vi "Oscilloscope_Analyzer.vi"(7 "Note":enum16{"Модулятор", "Команда", "Кадер", "Кодер"}(ring), 8 "error in (no error)":errorcluster, 11 "ISO 14443 A DOWN in":refnum<class "ISO 14443 A DOWN.lvclass">) -> (0 "error out":errorcluster, 3 "ISO 14443 A DOWN out":refnum<class "ISO 14443 A DOWN.lvclass">)   [LabVIEW 2019]
uses:
  ISO 14443 A DOWN.lvclass
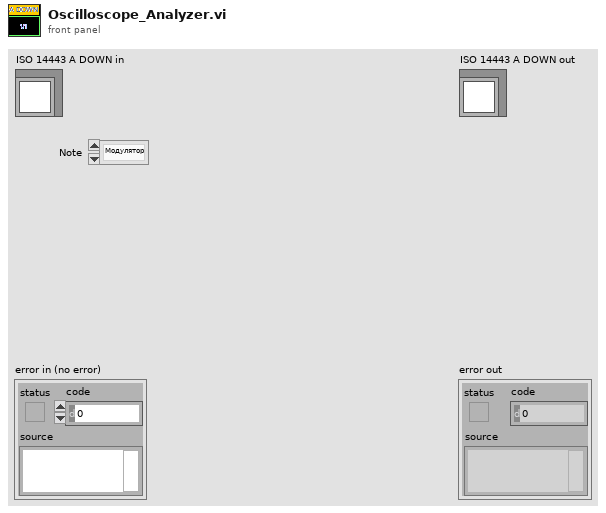
[diagram p1: front panel]
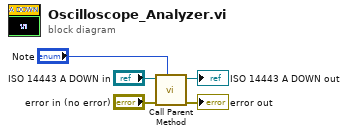
[diagram p0: block diagram]
diagram:
  n1 = call-parent "Call Parent Method"("Note"="Note", "error in (no error)"="error in (no error)", "RFID system in"="ISO 14443 A DOWN in") -> ("error out"=→"error out":errorcluster, "RFID system out"=→"ISO 14443 A DOWN out":refnum<class "ISO 14443 A DOWN.lvclass">)  [unwired: 7 in]
